vi "calculate new center voltage.vi"(8 "错误输入（无错误）":errorcluster, 9 "数据记录文件引用句柄":refnum<k1>, 10 "Original":T1 {"Zoom (V)" scale=0.0..1.0; "X Pos." scale=-2.0..2.0; "Y Pos." scale=-2.0..2.0}, 11 "CursLoc":cluster{"X":dbl, "Y":dbl}) -> (0 "错误输出":errorcluster, 2 "y pos (V)":dbl, 3 "x pos (V)":dbl)   [LabVIEW 2013]
uses:
  init & communication/Setting-User input.ctl
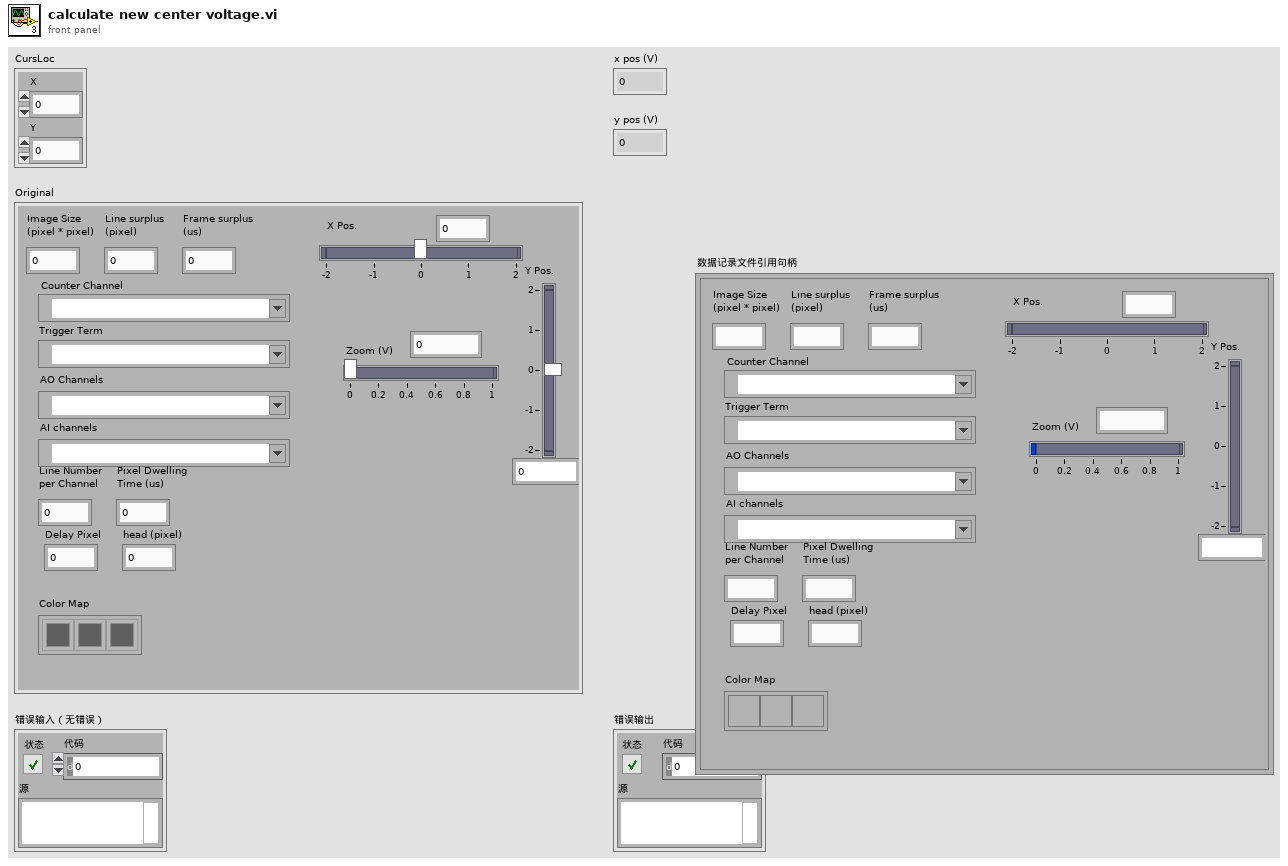
[diagram p1: front panel]
types:
  T1 = typedef "Setting-User input.ctl" = cluster{"Image Size\n(pixel * pixel)":i32, "Counter Channel":tag, "Trigger Term":tag, "AO Channels":tag, "Y Pos.":dbl, "X Pos.":dbl, "Line surplus\n(pixel)":i32, "Frame surplus\n(us)":i32, "AI channels":tag, "Line Number\nper Channel":i32, "Delay Pixel":i32, "Pixel Dwelling\nTime (us)":i32, "Color Map":u32[], "head (pixel)":i32, "Zoom (V)":dbl}
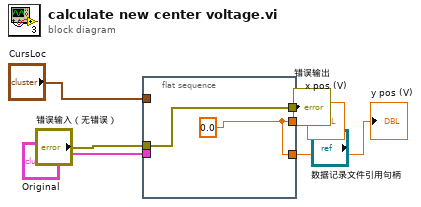
[diagram p0: block diagram]
diagram:
  n1 = flat-sequence {
    tunnel: "CursLoc" -> [_]
    tunnel: "Original" -> [_]
    tunnel: [w7] -> w3
    tunnel: "错误输入（无错误）" -> [w8]
    tunnel: [w8] -> w5
    tunnel: [w7] -> w6
    frame #0 {
      w7 = 0.0
    }
  }
  "y pos (V)" <- w6
  "错误输出" <- w5
  "x pos (V)" <- w3
